vi "conv_c_to_k.vi"(1 "deg. C":dbl) -> (0 "deg. K":dbl)   [LabVIEW 2023]
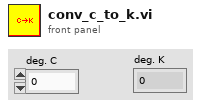
[diagram p1: front panel]
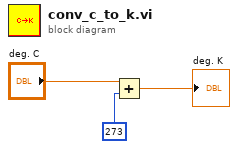
[diagram p0: block diagram]
diagram:
  n1 = Add(x="deg. C", y=273) -> (x+y=→"deg. K":dbl)
